vi "releaseRef.vi"(8 "error in (no error)":errorcluster, 11 "IBaseObject in":refnum<class "IBaseObject.lvclass">) -> (0 "error out":errorcluster)   [LabVIEW 2022 SP3, in "openDAQ.lvlib" / "IBaseObject.lvlib" / "IBaseObject.lvclass"]
uses:
  <instrlib>/openDAQ/Public/Classes/IBaseObject/IBaseObject.lvclass
  <instrlib>/openDAQ/Public/Classes/IBaseObject/IBaseObject.lvclass/IBaseObject.ctl
  <instrlib>/openDAQ/Binaries/Windows/x86/copendaq32.dll
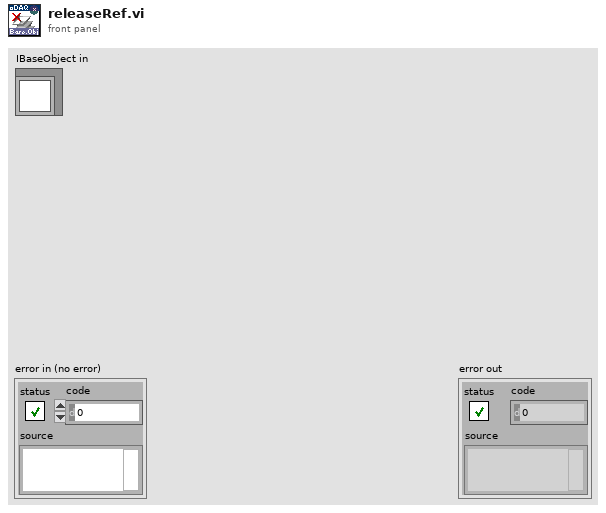
[diagram p1: front panel]
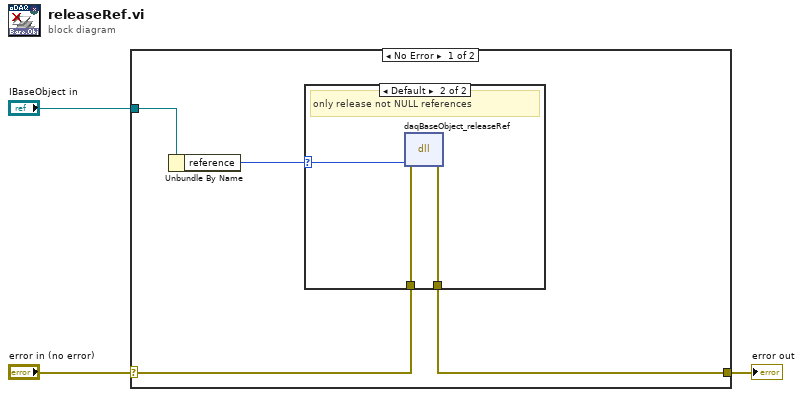
[diagram p0: block diagram]
diagram:
  n1 = case shown="No Error" "error in (no error)" {
    selector: "error in (no error)" -> [w6 w12]
    tunnel: [w5 w12] -> w2
    tunnel: "IBaseObject in" -> [w7 _]
    frame No Error {
      n2 = Unbundle By Name(w7) -> ("reference"=w4:i64)
      n3 = case shown="Default" w4 {
        selector: w4 -> [_ w9]
        tunnel: w6 -> [w8 w11]
        tunnel: [w8 w10] -> w5
        frame 0 {
        }
        frame Default {
          # "only release not NULL references"
          n4 = dll-call lib="C:/Program Files (x86)/National Instruments/LabVIEW 2022/instr.lib/openDAQ/Binaries/Windows/x86/copendaq*.*" fn="daqBaseObject_releaseRef"(error in=w11, "reference"=w9) -> (error out=w10:errorcluster)  [unwired: 4 in, 1 out]
        }
      }
    }
    frame Error {
    }
  }
  "error out" <- w2
